vi "Write Local Port.vi"(10 "local port":u16=2001, 11 "TCP Stream in":refnum<class "TCP Stream.lvclass">) -> (3 "TCP Stream out":refnum<class "TCP Stream.lvclass">)   [LabVIEW 2020, in "TCP Stream.lvclass"]
doc: "Use this VI to set the local port to be used for the stream connection."
uses:
  TCP Stream.lvclass
  TCP Stream.lvclass/TCP Stream.ctl
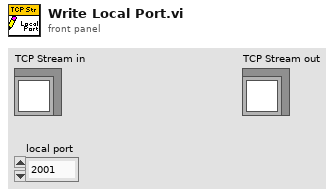
[diagram p1: front panel]
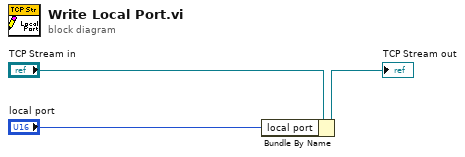
[diagram p0: block diagram]
diagram:
  n1 = Bundle By Name(cluster="TCP Stream in", "local port"="local port") -> (→"TCP Stream out":refnum<class "TCP Stream.lvclass">)
